vi "Untitled 1.vi"() -> ()   [LabVIEW 2014]
uses:
  C:/Projects/Serial Sectioning OCT/Software/Thorlabs.MotionControl.Controls.dll
  Thorlabs.MotionControl.Controls.dll
  C:/Projects/Serial Sectioning OCT/Software/Thorlabs.MotionControl.IntegratedStepperMotorsCLI.dll
  Thorlabs.MotionControl.IntegratedStepperMotorsCLI.dll
panel:
  out "Array 2":u32[](array[numeric])
  in  "LongTravelStageControl X":refnum<k24>(container)
  in  "Motion In":T1(array[cluster])=[{"LTS Ref"=refnum, "Device SN"="45876539", "Is.Connected?"=FALSE, "Is.Enabled?"=FALSE, "DevicePosition"=0.0}]
  out "Array":T1(array[cluster])
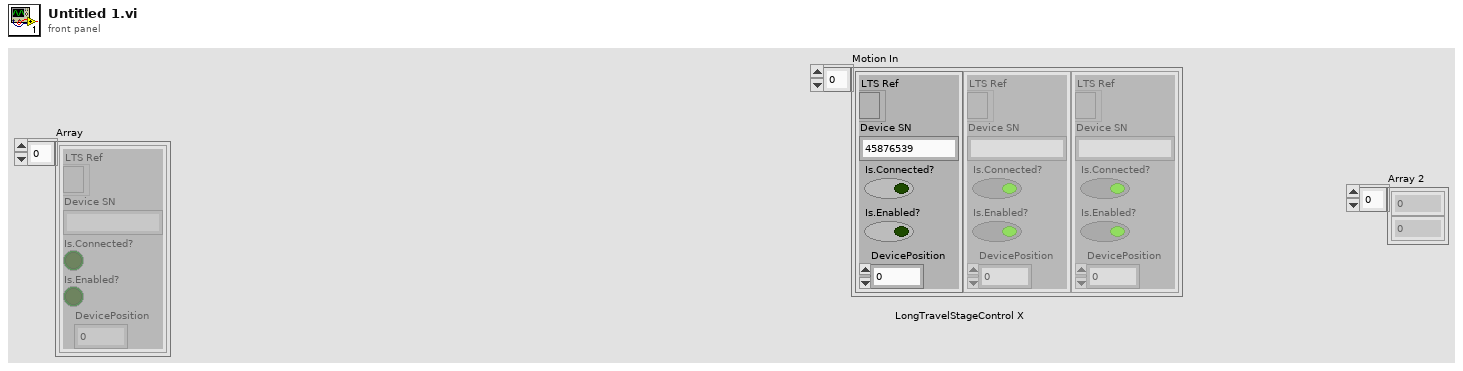
[diagram p1: front panel]
types:
  T1 = cluster{"LTS Ref":refnum<k24>, "Device SN":string, "Is.Connected?":bool, "Is.Enabled?":bool, "DevicePosition":dbl}[]
  T2 = cluster{"LTS Ref":refnum<k24>, "Device SN":string, "Is.Connected?":bool, "Is.Enabled?":bool, "DevicePosition":dbl}
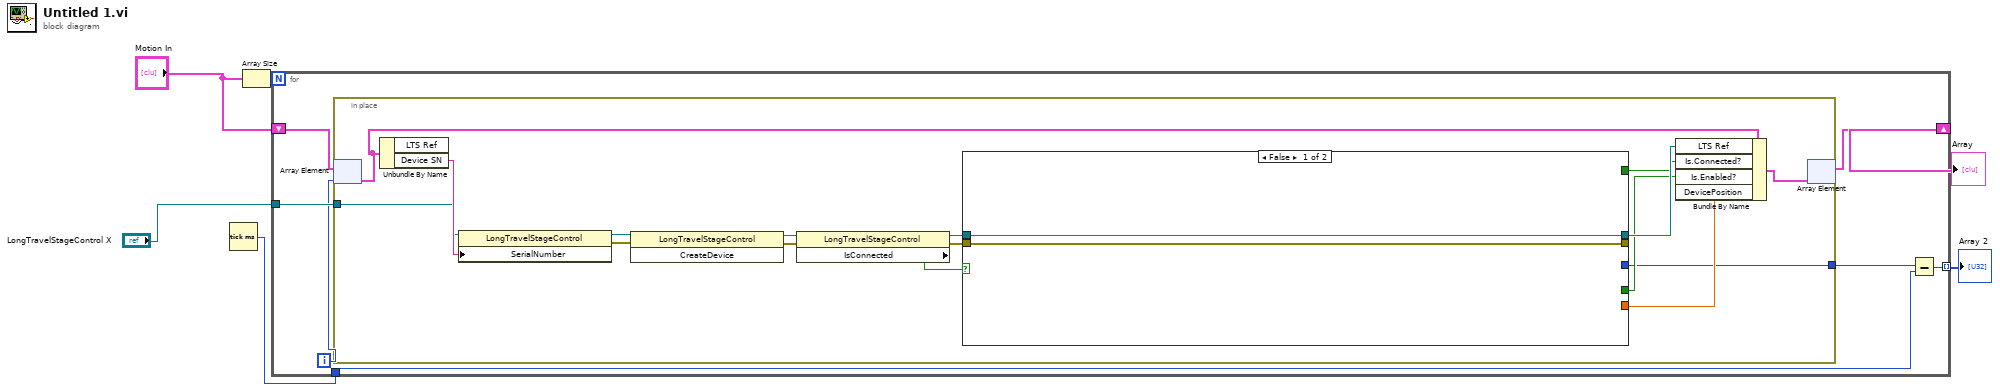
[diagram p0: block diagram]
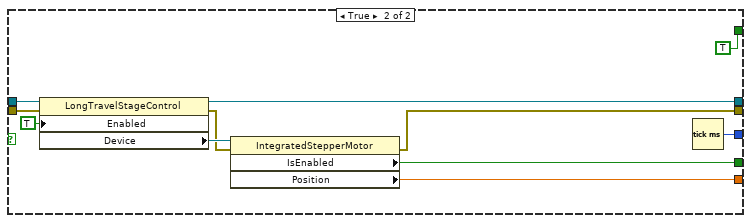
[diagram p2: hidden frame]
diagram:
  n1 = Tick Count (ms)() -> (millisecond timer value=w3:u32)
  n2 = Array Size(array="Motion In") -> (size(s)=w4:i32)
  n3 = for {
    N: w4 -> [_]
    tunnel: "LongTravelStageControl X" -> [w13]
    shift-right: [w10] -> w6
    shift-left: "Motion In" -> [w12]
    tunnel: w3 -> [w8]
    tunnel: [w7] -> w1 mode=indexing
    i -> [w11]
    n4 = in-place {
      in-place-border: w13 -> [w17]
      in-place-border: [w14] -> w9
      n5 = in-place-array #1(w12, w11) -> (w16:T2)
      n6 = Unbundle By Name(w16) -> ("Device SN"=w29:string)  [unwired: 1 out]
      n7 = property class="LongTravelStageControl"(reference=w17, "SerialNumber"=w29) -> (reference out=w28:refnum<k24>, error out=w27:errorcluster)  [unwired: 1 in]
      n8 = invoke class="LongTravelStageControl" method="CreateDevice"(reference=w28, error in=w27) -> (reference out=w26:refnum<k24>, error out=w25:errorcluster)  [unwired: 1 in, 1 out]
      n9 = property class="LongTravelStageControl"(reference=w26, error in=w25) -> (reference out=w23:refnum<k24>, error out=w22:errorcluster, "IsConnected"=w24:bool)
      n10 = case shown="False" w24 {
        tunnel: w23 -> [w30 w42]
        tunnel: w22 -> [w31 w41]
        tunnel: [w31 w35] -> _
        tunnel: [w30 w37] -> w21
        tunnel: [_ w39] -> w19
        tunnel: [_ w34] -> w18
        tunnel: [_ TRUE ("Enabled")] -> w20
        tunnel: [_ w32] -> w14
        frame False {
        }
        frame True {
          n11 = property class="LongTravelStageControl"(reference=w42, error in=w41, "Enabled"=TRUE) -> (reference out=w37:refnum<k24>, error out=w36:errorcluster, "Device"=w38:refnum<k24>)
          n12 = property class="IntegratedStepperMotor"(reference=w38, error in=w36) -> (error out=w35:errorcluster, "IsEnabled"=w39:bool, "Position"=w34:dbl)  [unwired: 1 out]
          n13 = Tick Count (ms)() -> (millisecond timer value=w32:u32)
        }
      }
      n14 = Bundle By Name(cluster=w16, "LTS Ref"=w21, "Is.Connected?"=w20, "Is.Enabled?"=w19, "DevicePosition"=w18) -> (w15:T2)
      n15 = in-place-array #1(w15) -> (w10:T1)  [unwired: 1 out]
    }
    n16 = Subtract(x=w9, y=w8) -> (x-y=w7:u32)
  }
  "Array" <- w6
  "Array 2" <- w1
